vi "路经检测与创建.vi"() -> (1 "错误音效文件":path, 2 "完成音效文件":path, 3 "通信配置文件路径":path)   [LabVIEW 2013]
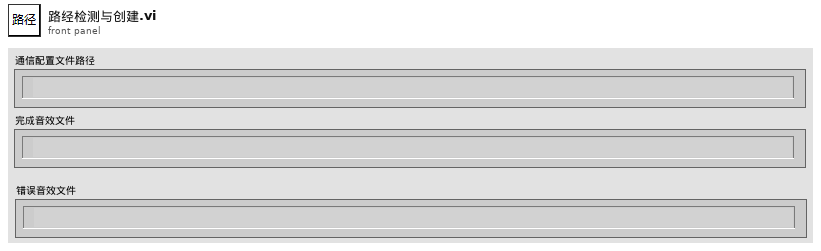
[diagram p1: front panel]
types:
  T1 = enum16{"open", "replace", "create", "open or create", "replace or create", "replace or create with confirmation"}
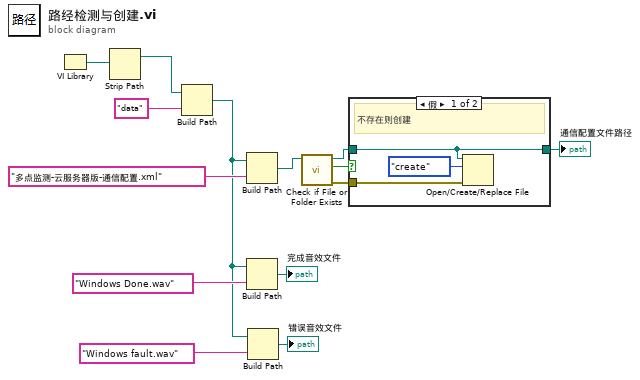
[diagram p0: block diagram]
diagram:
  n1 = VI Library() -> (path=w11:path)
  n2 = Strip Path(path=w11) -> (stripped path=w14:path)  [unwired: 1 out]
  n3 = Build Path(base path=w14, name or relative path="data" ("名称或相对路径")) -> (appended path=w1:path)
  n4 = Build Path(base path=w1, name or relative path="多点监测-云服务器版-通信配置.xml" ("名称或相对路径")) -> (appended path=w7:path)
  n5 = Build Path(base path=w1, name or relative path="Windows Done.wav" ("名称或相对路径")) -> (appended path=→"完成音效文件":path)
  n6 = Build Path(base path=w1, name or relative path="Windows fault.wav" ("名称或相对路径")) -> (appended path=→"错误音效文件":path)
  n7 = call <vilib>:"Check if File or Folder Exists.vi"("path"=w7) -> ("error out"=w10:errorcluster, "file or folder exists?"=w8:bool, "dup path"=w9:path)  [unwired: 8 in]
  n8 = case shown="假" w8 {
    tunnel: w10 -> [w16 _]
    tunnel: w9 -> [w15 w18]
    tunnel: [w15 w18] -> w6
    frame False {
      # "不存在则创建"
      n9 = Open/Create/Replace File(file path (use dialog)=w15, error in=w16, operation (0:open)=T1."create" ("操作(0:open)")) -> ()  [unwired: 3 in, 3 out]
    }
    frame True {
      # "存在则输出"
    }
  }
  "通信配置文件路径" <- w6
